vi "Read Payload.vi"(8 "error in (no error)":errorcluster, 9 "Payload Size":u16, 11 "IP Connection in":refnum<class "IP Connection.lvclass">) -> (0 "error out":errorcluster, 2 "Data":string, 3 "IP Connection out":refnum<class "IP Connection.lvclass">)   [LabVIEW 2011, in "Tinkerforge.lvlib" / "IP Connection.lvclass"]
doc: "This VI reads the given number of data bytes."
uses:
  IP Connection.lvclass
  IP Connection.lvclass/IP Connection.ctl
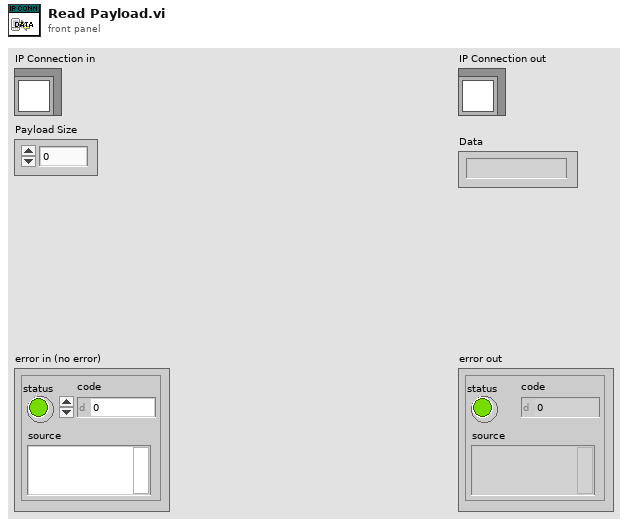
[diagram p1: front panel]
types:
  T1 = enum16{"Standard", "Buffered", "CRLF", "Immediate"}
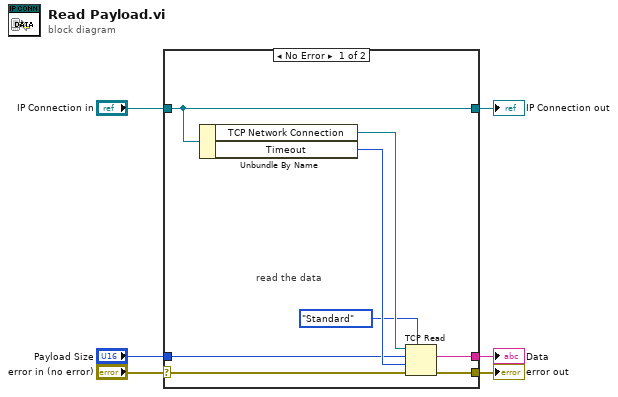
[diagram p0: block diagram]
diagram:
  n1 = case shown="No Error" "error in (no error)" {
    selector: "error in (no error)" -> [w13 w16]
    tunnel: [w12 w16] -> w5
    tunnel: [w14 w15] -> w3
    tunnel: "IP Connection in" -> [w14 w15]
    tunnel: "Payload Size" -> [w8 _]
    tunnel: [w7 _] -> w1
    frame No Error {
      # "read the data"
      n2 = Unbundle By Name(w14) -> ("TCP Network Connection"=w11:refnum<k5>, "Timeout"=w10:i32)
      n3 = TCP Read(connection ID=w11, bytes to read=w8, error in (no error)=w13, 7:T1."Standard" ("mode (standard)"), 9:w10) -> (data out=w7:string, error out=w12:errorcluster)  [unwired: 1 out]
    }
    frame Error {
    }
  }
  "error out" <- w5
  "IP Connection out" <- w3
  "Data" <- w1
